vi "Destroy to SFTP File.vi"(8 "Error In":errorcluster, 10 "SFTP Attributes":refnum<class "SFTP Attributes.lvclass">, 11 "SFTP File In":refnum<class "SFTP File.lvclass">) -> (0 "Error Out":errorcluster, 3 "SFTP File Out":refnum<class "SFTP File.lvclass">)   [LabVIEW 2021, in "Field_RnD_Services_LIBSSH2_Toolkit.lvlib" / "SFTP Attributes.lvclass"]
doc: "Passes through the SFTP File object and destroys the associated SFTP Attributes object."
uses:
  SFTP Attributes.lvclass
  SFTP File/SFTP File.lvclass
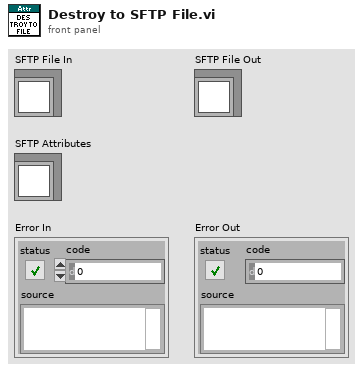
[diagram p1: front panel]
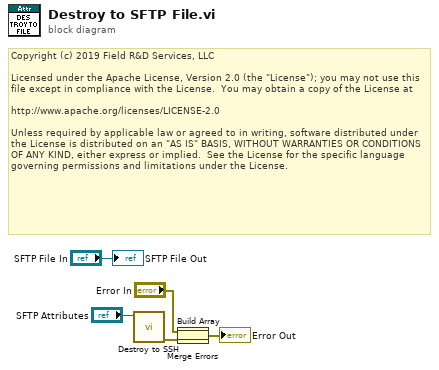
[diagram p0: block diagram]
diagram:
  # "Copyright (c) 2019 Field R&D Services, LLC\n\nLicensed under the Apache License, Version 2.0 (the \"License\"); you may not use this file except in compliance with the License.  You may obtain a copy of the License at\n\nhttp://www.apache.org/licenses/LICENSE-2.0\n\nUnless required by applicable law or agreed to in writing, software distributed under the License is distributed on an \"AS IS\" BASIS, WITHOUT WARRANTIES OR CONDITIONS OF ANY KIND, either express or implied.  See the License for the specific language governing permissions and limitations under the License."
  n1 = call "Destroy to SSH.vi"("SFTP Attributes"="SFTP Attributes") -> ("Error Out"=w3:errorcluster)  [unwired: 9 in, 1 out]
  n2 = Build Array("Error In", w3) -> (w1:errorcluster[])
  n3 = Merge Errors(w1) -> (→"Error Out":errorcluster)
  "SFTP File Out" <- "SFTP File In"
